vi "题目5.vi"() -> ()   [LabVIEW 2017]
panel:
  out "显示面板":T1 {"转速（r/s）" scale=0.0..8000.0; "速度（km/h）" scale=0.0..300.0; "油量" scale=0.0..200.0 scale format="%.3f"}
  in  "停止":bool
  in  "控制面板":T2 {"档位" scale=0.0..6.0; "油门" scale=0.0..10.0}
  out "油量报警":bool
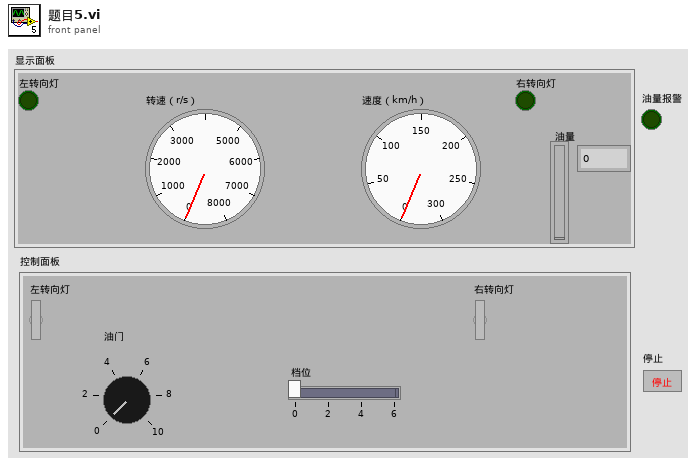
[diagram p1: front panel]
types:
  T1 = cluster{"左转向灯":bool, "右转向灯":bool, "转速（r/s）":dbl, "速度（km/h）":dbl, "油量":dbl}
  T2 = cluster{"左转向灯":bool, "右转向灯":bool, "油门":dbl, "档位":dbl}
  T3 = cluster{"左转向灯":bool, "右转向灯":bool, dbl, dbl, "y":dbl}
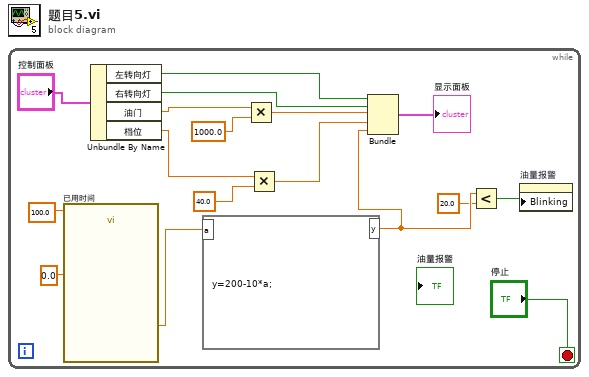
[diagram p0: block diagram]
diagram:
  n1 = while {
    stop <- "停止" stop-if-true
    n2 = call "已用时间"("Time Target (s)"=100.0, "Set Start Time (s)"=0.0) -> ("Elapsed Time (s)"=w1:dbl)  [unwired: 10 in, 7 out]
    n3 = Unbundle By Name("控制面板") -> ("左转向灯"=w12:bool, "右转向灯"=w11:bool, "油门"=w17:dbl, "档位"=w15:dbl)
    n4 = formula code="y=200-10*a;"("a"=w1) -> ("y"=w7:dbl)
    n5 = Multiply(x=w17, y=1000.0) -> (x*y=w10:dbl)
    n6 = Multiply(x=w15, y=40.0) -> (x*y=w9:dbl)
    n7 = Bundle("左转向灯"=w12, "右转向灯"=w11, w10, w9, "y"=w7) -> (→"显示面板":T3)  [unwired: 1 in]
    n8 = Less?(x=w7, y=20.0) -> (x < y?=w5:bool)
    n9 = property on="油量报警" class="Bool (严格)"("Blinking"=w5) -> ()  [unwired: 2 in, 2 out]
  }
